vi "ElevatorSim_SetState.vi"(9 "System State":T1, 11 "in ElevatorSim":T2 {"GearBox"."Jr_KgM2" format="%13.5p"; "GearBox"."L_H" format="%13.5p"; "GearBox"."Kt_NMPerAmp" format="%13.5p"; "GearBox"."KvINV_RadPerSecPerVolt" format="%13.5p"; "GearBox"."R_Ohms" format="%13.5p"; "GearBox"."FreeSpeed_RadPerSec" format="%13.5p"; "GearBox"."FreeCurrent_Amps" format="%13.5p"; "GearBox"."StallCurrent_Amps" format="%13.5p"; "GearBox"."StallTorque_NM" format="%13.5p"; "GearBox"."nominalVoltage_Volts" format="%13.5p"}) -> (0 "Size Coerced":bool, 3 "out ElevatorSim":T2 {"GearBox"."Jr_KgM2" format="%13.5p"; "GearBox"."L_H" format="%13.5p"; "GearBox"."Kt_NMPerAmp" format="%13.5p"; "GearBox"."KvINV_RadPerSecPerVolt" format="%13.5p"; "GearBox"."R_Ohms" format="%13.5p"; "GearBox"."FreeSpeed_RadPerSec" format="%13.5p"; "GearBox"."FreeCurrent_Amps" format="%13.5p"; "GearBox"."StallCurrent_Amps" format="%13.5p"; "GearBox"."StallTorque_NM" format="%13.5p"; "GearBox"."nominalVoltage_Volts" format="%13.5p"})   [LabVIEW 2019, in "Trajectory_Library.lvlib"]
doc: "Sets the system state.\n \nInputs:\n - ElevatorSim -- Data cluster\n - state -- The new state.\n\nOutputs:\n - OutElevatorSim -- Updated data cluster\n - SizeCoerced -- If TRUE, an error occured. Execution may continue."
uses:
  Trajectory_Library.lvlib
  ELEVATOR_SIM.ctl
  LINEAR_SYSTEM_SIM.ctl
  LINEAR_SYSTEM.ctl
  <vilib>/Analysis/Matrix/Datatypes/RealMatrix.ctl
  DCMOTOR.CTL
  MatBuilder_Create.vi
  <vilib>/Analysis/Matrix/NI_Matrix.lvlib
panel:
  # "<States, 1>"
  # "<Outputs, 1>"
  # "<Inputs, 1>"
  # "<Outputs, 1>"
  # "<States,States>"
  # "<States,Inputs>"
  # "<Outputs,States>"
  # "<Outputs,Inputs>"
  # "<States, 1>"
  # "<Outputs, 1>"
  # "<Inputs, 1>"
  # "<Outputs, 1>"
  # "<States,States>"
  # "<States,Inputs>"
  # "<Outputs,States>"
  # "<Outputs,Inputs>"
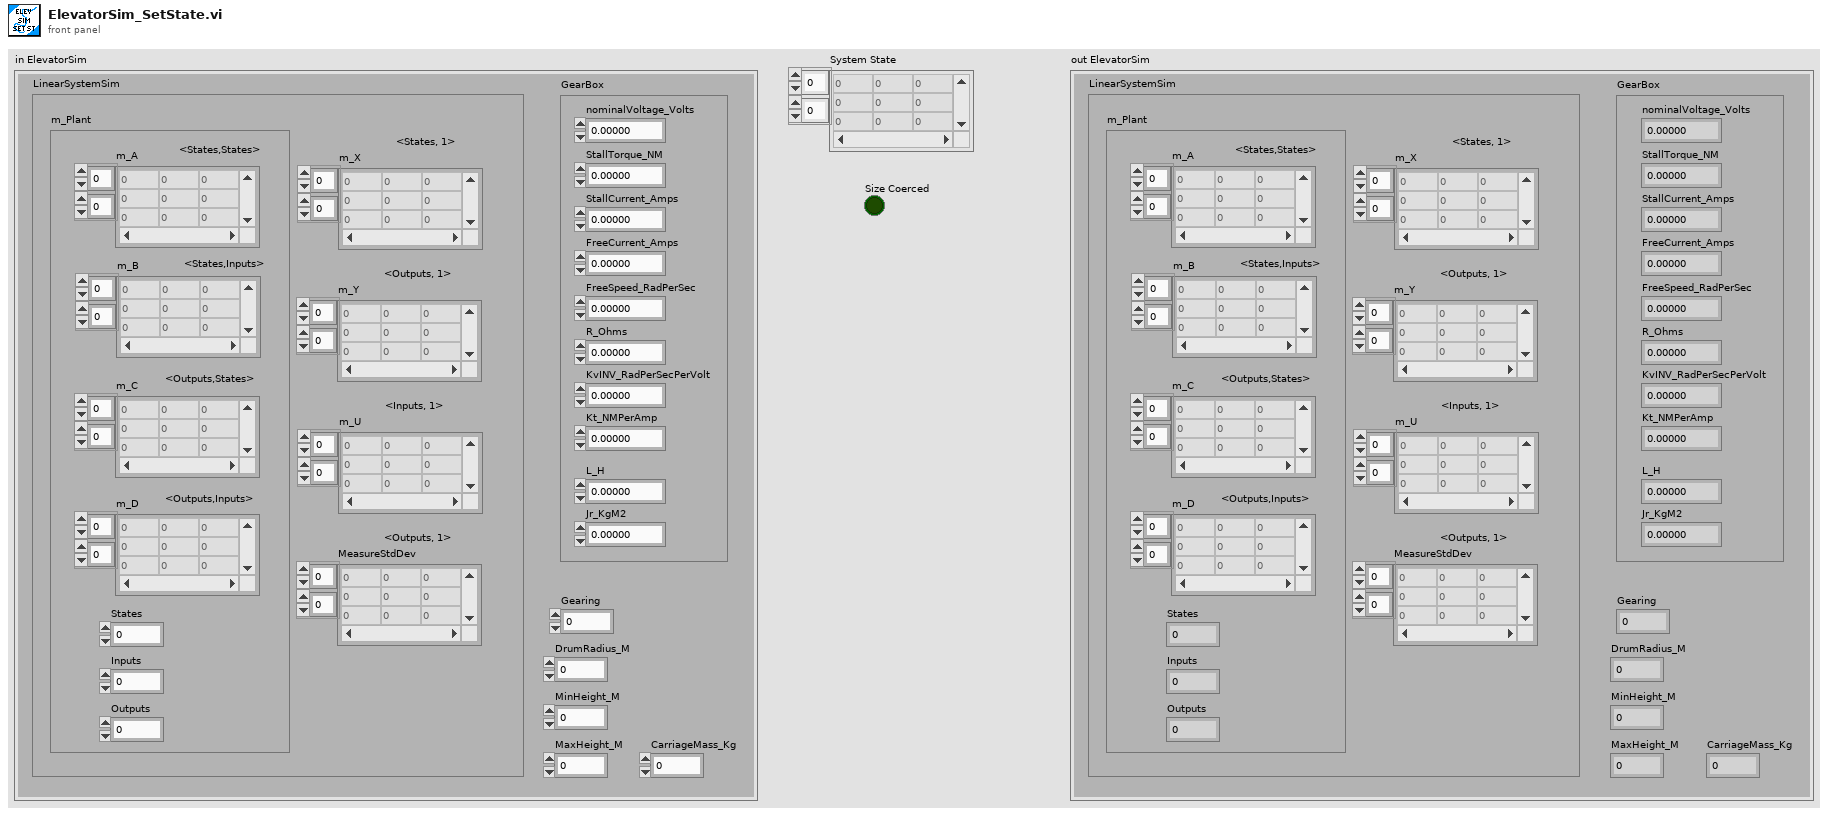
[diagram p1: front panel]
types:
  T1 = typedef "NI_Matrix.lvlib/RealMatrix.ctl" = dbl[][]
  T2 = typedef "Trajectory_Library.lvlib/ELEVATOR_SIM.ctl" = cluster{"LinearSystemSim":T3, "GearBox":T5, "Gearing":dbl, "DrumRadius_M":dbl, "MinHeight_M":dbl, "MaxHeight_M":dbl, "CarriageMass_Kg":dbl}
  T3 = typedef "Trajectory_Library.lvlib/LINEAR_SYSTEM_SIM.ctl" = cluster{"m_Plant":T4, "m_X":T1, "m_Y":T1, "m_U":T1, "MeasureStdDev":T1}
  T4 = typedef "Trajectory_Library.lvlib/LINEAR_SYSTEM.ctl" = cluster{"m_A":T1, "m_B":T1, "m_C":T1, "m_D":T1, "States":i32, "Inputs":i32, "Outputs":i32}
  T5 = typedef "Trajectory_Library.lvlib/DCMOTOR.CTL" = cluster{"nominalVoltage_Volts":dbl, "StallTorque_NM":dbl, "StallCurrent_Amps":dbl, "FreeCurrent_Amps":dbl, "FreeSpeed_RadPerSec":dbl, "R_Ohms":dbl, "KvINV_RadPerSecPerVolt":dbl, "Kt_NMPerAmp":dbl, "L_H":dbl, "Jr_KgM2":dbl}
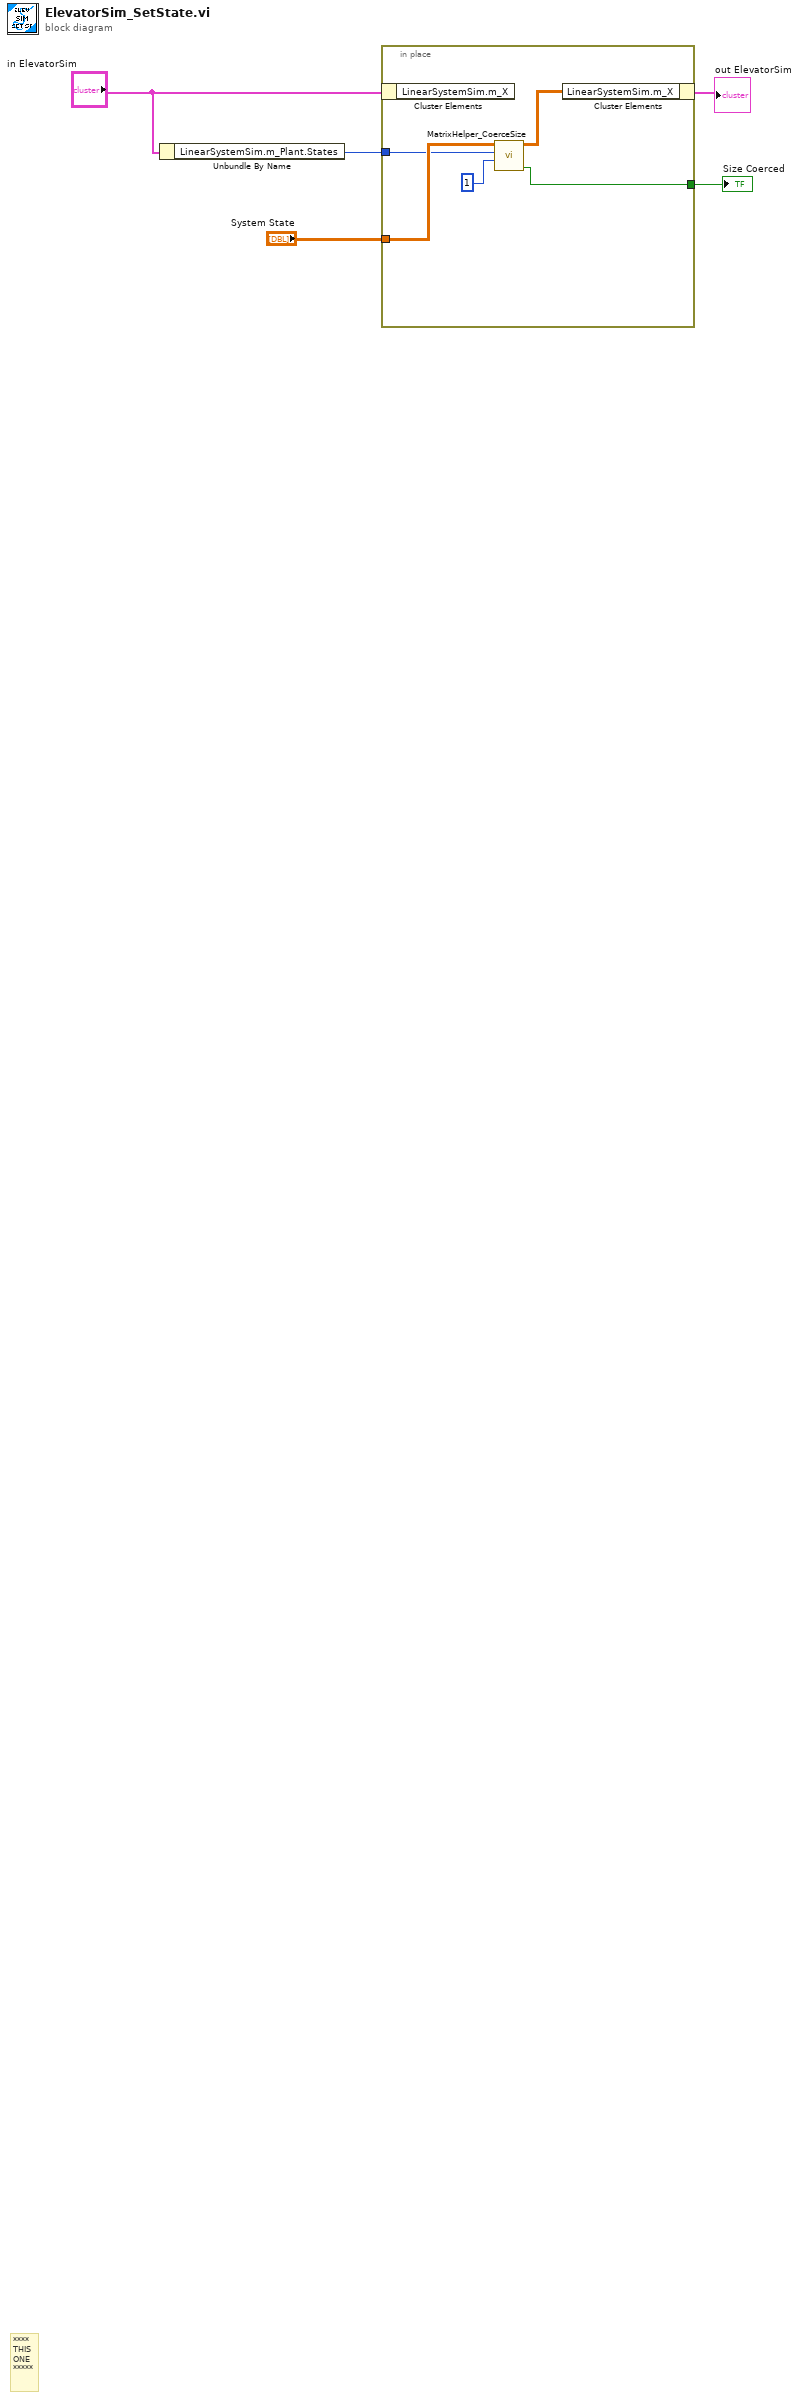
[diagram p0: block diagram]
diagram:
  # "****\nTHIS\nONE\n*****"
  n1 = Unbundle By Name("in ElevatorSim") -> ("LinearSystemSim.m_Plant.States"=w2:i32)
  n2 = in-place {
    in-place-border: "System State" -> [w10]
    in-place-border: w2 -> [w8]
    in-place-border: [w6] -> w1
    n3 = in-place-cluster #1("in ElevatorSim") -> ()  [unwired: 1 out]
    n4 = call "MatrixHelper_CoerceSize.vi"("Columns"=1, "Rows"=w8, "input matrix"=w10) -> ("Coerced"=w6:bool, "output matrix"=w7:T1)  [unwired: 7 in]
    n5 = in-place-cluster #1("LinearSystemSim.m_X"=w7) -> (→"out ElevatorSim":T2)
  }
  "Size Coerced" <- w1
